vi "3.vonversion_continious_to_Binary.vi"() -> ()   [LabVIEW 2018]
uses:
  <vilib>/Waveform/DWDTOps.llb/DWDT Analog to Digital.vi
  <vilib>/Waveform/DTblOps.llb/DTbl Digital to Binary U32.vi
  <vilib>/measure/NI_MABase.lvlib
panel:
  in  "Stop Button":bool
  out "frequence Echantio":dbl=1000.0
  in  "resolution":dbl=4.0
  out "Waveform Graph 3":waveform(dbl)(graph)
  out "Waveform Graph 2":waveform(dbl)[](graph)
  out "Waveform Graph":waveform(dbl)(graph)
  in  "Frequence":dbl=3.0
  in  "Amplitude":dbl=1.0
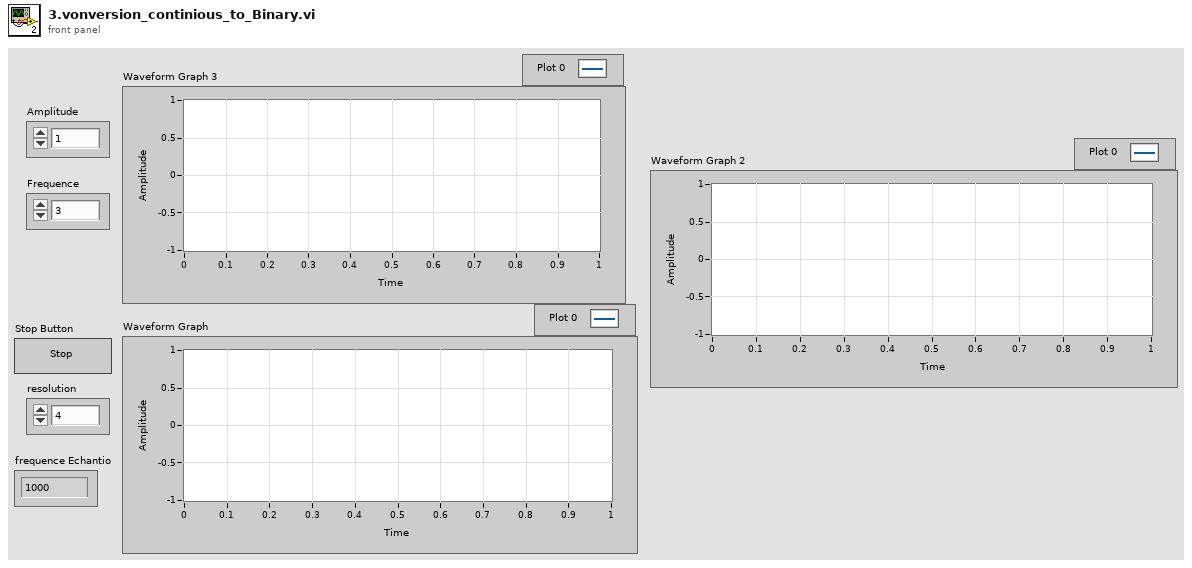
[diagram p1: front panel]
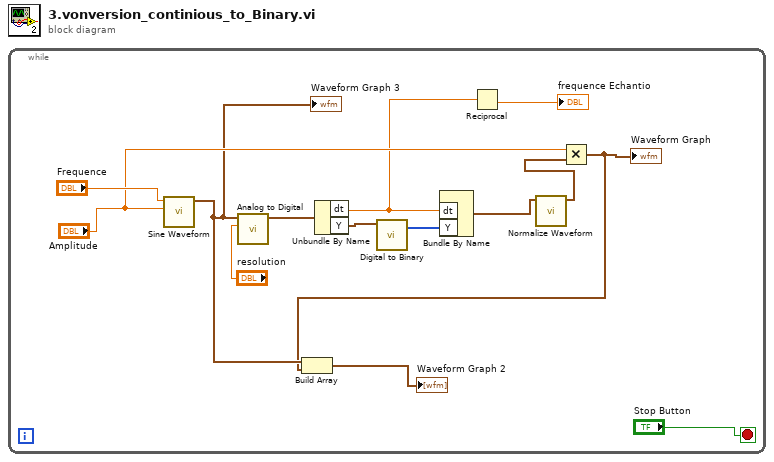
[diagram p0: block diagram]
diagram:
  n1 = while {
    stop <- "Stop Button" stop-if-true
    n2 = call <vilib>:"Sine Waveform.vi"("amplitude"="Amplitude", "frequency"="Frequence") -> ("signal out"=w7:waveform(dbl))  [unwired: 8 in, 1 out]
    "Waveform Graph 3" <- w7
    n3 = call-poly <vilib>:"Analog to Digital.vi"("resolution (16 bit)"="resolution", "analog waveform"=w7) -> ("digital waveform"=w12:digitalwaveform)  [unwired: 6 in, 3 out]
    n4 = Unbundle By Name(w12) -> ("dt"=w4:dbl, "Y"=w14:digitaldata)
    n5 = call-poly <vilib>:"Digital to Binary.vi"("digital data"=w14) -> ("binary array"=w13:u32[])  [unwired: 9 in, 1 out]
    n6 = Bundle By Name("dt"=w4, "Y"=w13) -> (w10:waveform(u32))  [unwired: 1 in]
    n7 = Reciprocal(x=w4) -> (1/x=→"frequence Echantio":dbl)
    n8 = call <vilib>:"Normalize Waveform.vi"("waveform in"=w10) -> ("normalized waveform"=w2:waveform(dbl))  [unwired: 7 in, 3 out]
    n9 = Multiply(x="Amplitude", y=w2) -> (x*y=w6:waveform(dbl))
    "Waveform Graph" <- w6
    n10 = Build Array(w7, w6) -> (→"Waveform Graph 2":waveform(dbl)[])
  }
